vi "LeftAndRight.vi"(9 "Left or Right":string, 10 "RobotDriveDevRef":T1, 11 "Duration (Seconds)":dbl) -> ()   [LabVIEW 2019]
uses:
  <vilib>/Rock Robotics/WPI/RobotDrive/WPI_RobotDriveDevRef.ctl
  <vilib>/Rock Robotics/WPI/MotorControl/WPI_MotorControlDeviceRef.ctl
  <vilib>/Rock Robotics/WPI/MotorControl/WPI_MotorControlType.ctl
  <vilib>/Rock Robotics/SystemInterfaces/DIO/FPGA_DIOPWMChannel.ctl
  <vilib>/Rock Robotics/WPI/PWM/WPI_PWMDeadband.ctl
  <vilib>/Rock Robotics/SystemInterfaces/DIO/FPGA_DIOChannel.ctl
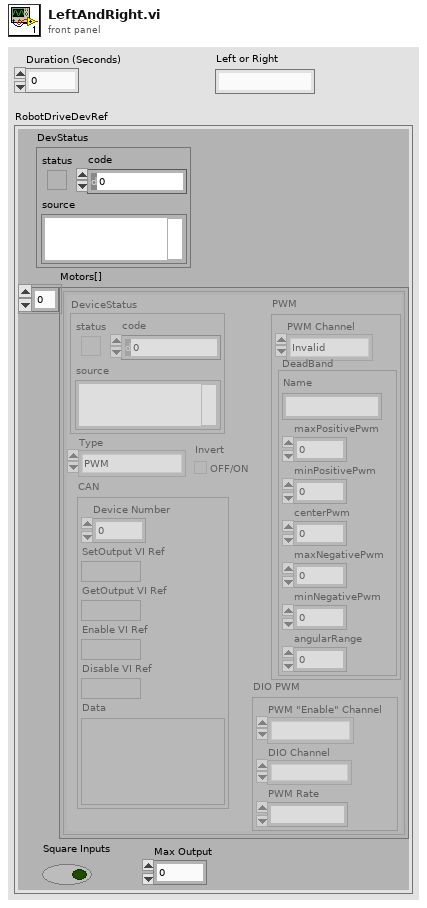
[diagram p1: front panel]
types:
  T1 = typedef "WPI_RobotDriveDevRef.ctl" = cluster{"DevStatus":errorcluster, "Motors[]":T2[], "Square Inputs":bool, "Max Output":dbl}
  T2 = typedef "WPI_MotorControlDeviceRef.ctl" = cluster{"DeviceStatus":errorcluster, "Type":T3, "PWM":cluster{"PWM Channel":T4, "DeadBand":T5}, "CAN":cluster{"Device Number":u8, "SetOutput VI Ref":variant, "GetOutput VI Ref":variant, "Enable VI Ref":variant, "Disable VI Ref":variant, "Data":variant}, "Invert":bool, "DIO PWM":cluster{"PWM \"Enable\" Channel":T4, "DIOChannel":T6, "PWM Rate":dbl}}
  T3 = typedef "WPI_MotorControlType.ctl" = enum16{"PWM", "CAN", "DIO PWM"}
  T4 = typedef "FPGA_DIOPWMChannel.ctl" = enum8{"PWM 0", "PWM 1", "PWM 2", "PWM 3", "PWM 4", "PWM 5", "PWM 6", "PWM 7", "PWM 8", "PWM 9", "PWM MXP 0", "PWM MXP 1", "PWM MXP 2", "PWM MXP 3", "PWM MXP 4", "PWM MXP 5", "PWM MXP 6", "PWM MXP 7", "PWM MXP 8", "PWM MXP 9", "Invalid"}
  T5 = typedef "WPI_PWMDeadband.ctl" = cluster{"Name":string, "maxPositivePwm":i32, "minPositivePwm":i32, "centerPwm":i32, "maxNegativePwm":i32, "minNegativePwm":i32, "angularRange":u16}
  T6 = typedef "FPGA_DIOChannel.ctl" = enum8{"DIO 0", "DIO 1", "DIO 2", "DIO 3", "DIO 4", "DIO 5", "DIO 6", "DIO 7", "DIO 8", "DIO 9", "DIO MXP 0", "DIO MXP 1", "DIO MXP 2", "DIO MXP 3", "DIO MXP 4", "DIO MXP 5", "DIO MXP 6", "DIO MXP 7", "DIO MXP 8", "DIO MXP 9", "DIO MXP 10", "DIO MXP 11", "DIO MXP 12", "DIO MXP 13", "DIO MXP 14", "DIO MXP 15", "SPI Port CS1", "SPI Port CS2", "SPI Port CS3", "SPI Port MISO", "SPI Port MOSI", "Invalid"}
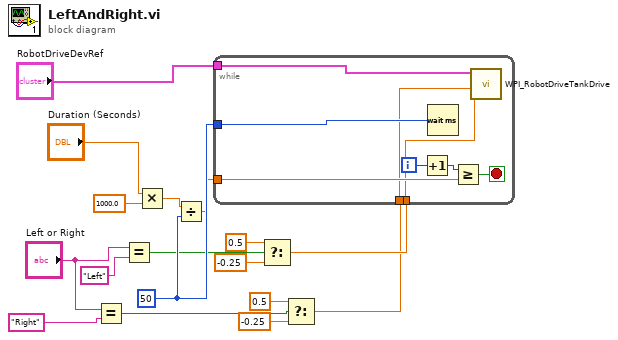
[diagram p0: block diagram]
diagram:
  w17 = 50
  n1 = Equal?(x="Left or Right", y="Right") -> (x = y?=w2:bool)
  n2 = Equal?(x="Left or Right", y="Left") -> (x = y?=w10:bool)
  n3 = Multiply(x="Duration (Seconds)", y=1000.0) -> (x*y=w15:dbl)
  n4 = Divide(x=w15, y=w17) -> (x/y=w16:dbl)
  n5 = Select(t=0.5, s=w10, f=-0.25) -> (s? t:f=w7:dbl)
  n6 = Select(t=0.5, s=w2, f=-0.25) -> (s? t:f=w1:dbl)
  n7 = while {
    tunnel: "RobotDriveDevRef" -> [w25]
    tunnel: w16 -> [w23]
    tunnel: w17 -> [w21]
    tunnel: w7 -> [w19]
    tunnel: w1 -> [w18]
    i -> [w24]
    stop <- w20 stop-if-true
    n8 = Increment(x=w24) -> (x+1=w22:i32)
    n9 = Wait (ms)(milliseconds to wait=w21) -> ()  [unwired: 1 out]
    n10 = Greater Or Equal?(x=w22, y=w23) -> (x >= y?=w20:bool)
    n11 = call <vilib>:"WPI_RobotDriveTankDrive.vi"("Right axis value"=w18, "Left axis value"=w19, "RobotDriveDevRef"=w25) -> ()  [unwired: 6 in, 3 out]
  }
